vi "Initialize.vi"(8 "error in":errorcluster, 10 "parameters":variant, 11 "node in":refnum<class "BuckBoost editor node.lvclass">) -> (0 "error out":errorcluster, 2 "summary":T2[](array[typedef]), 3 "data value reference":T1)   [LabVIEW 2017, in "BuckBoost editor node.lvclass"]
doc: "Initializes the data of a node to its default state.\nThe object is not created inside of this VI, because it is created from a File depending on user selection."
uses:
  BuckBoost editor node.lvclass
  C:/Program Files (x86)/National Instruments/LabVIEW 2017/vi.lib/NI/Configuration Framework/Node/NISE_CEF_Node.lvclass
  <vilib>/NI/Configuration Framework/Node/Summary.ctl
  <vilib>/NI/Configuration Framework/Node/NodeRef.ctl
  <vilib>/NI/Configuration Framework/Node/NISE_CEF_Node.lvclass
  module/configuration/BuckBoost configuration.lvclass
  C:/Program Files (x86)/National Instruments/LabVIEW 2017/vi.lib/NI/Configuration Framework/serializable configuration/NISE_CEF_serializable configuration.lvclass
  <vilib>/NI/PowerElectronicsControl/Buck-Boost/RealTime/modulationConfig.ctl
  <vilib>/NI/PowerElectronicsControl/Buck-Boost/RealTime/TuningParameters.ctl
  <vilib>/rvi/Analysis/control/PID/Typedef/niFpgaPID_PIGains.ctl
  <vilib>/NI/PowerElectronicsControl/Buck-Boost/FPGA/contState.ctl
  module/configuration/BuckBoost configuration.lvclass/BuckBoost configuration.ctl
  module/configuration/Write numOfInterleaves.vi
  module/configuration/Write TuningParameters.vi
  module/configuration/Write modulationConfig.vi
  <vilib>/NI/DCAF/Tag Editor Core/control module/editor node/control module editor.lvclass
  <vilib>/NI/Configuration Framework/serializable configuration/NISE_CEF_serializable configuration.lvclass
  <vilib>/NI/PowerElectronicsControl/Buck-Boost/RealTime/BuckBoostInterface.lvlib
  <vilib>/NI/PowerElectronicsControl/Buck-Boost/FPGA/BuckBoost.lvlib
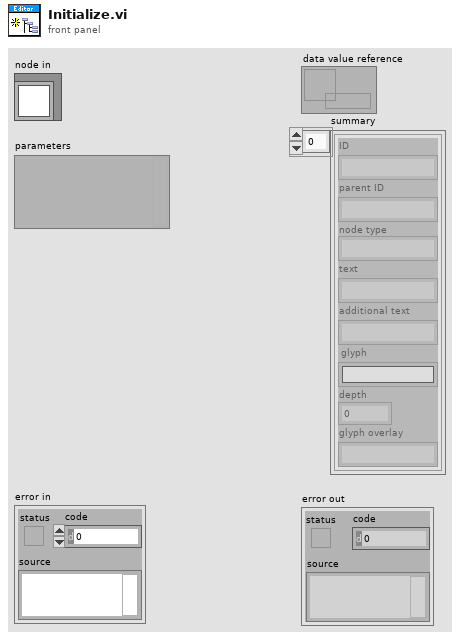
[diagram p1: front panel]
types:
  T1 = typedef "NISE_CEF_Node.lvclass/NodeRef.ctl" = refnum<data-value>
  T2 = typedef "NISE_CEF_Node.lvclass/Summary.ctl" = cluster{"ID":string, "parent ID":string, "node type":string, "text":string, "additional text":string, "glyph":string, "depth":i32, "glyph overlay":string}
  T3 = typedef "BuckBoostInterface.lvlib/TuningParameters.ctl" = cluster{"gains":T4, "manualInput":sgl, "rampRate":sgl, "pertAmp":sgl, "pertFreq":sgl, "controlFreq":sgl, "state":T5}
  T4 = typedef "niFpgaPID_PIGains.ctl" = cluster{"proportional gain":sgl, "integral gain":sgl}
  T5 = typedef "BuckBoost.lvlib/contState.ctl" = enum16{"disabled", "manual", "normal", "perturb"}
  T6 = typedef "BuckBoostInterface.lvlib/modulationConfig.ctl" = cluster{"SwitchingSpeed":dbl, "Deadband":dbl, "modulationRate":dbl}
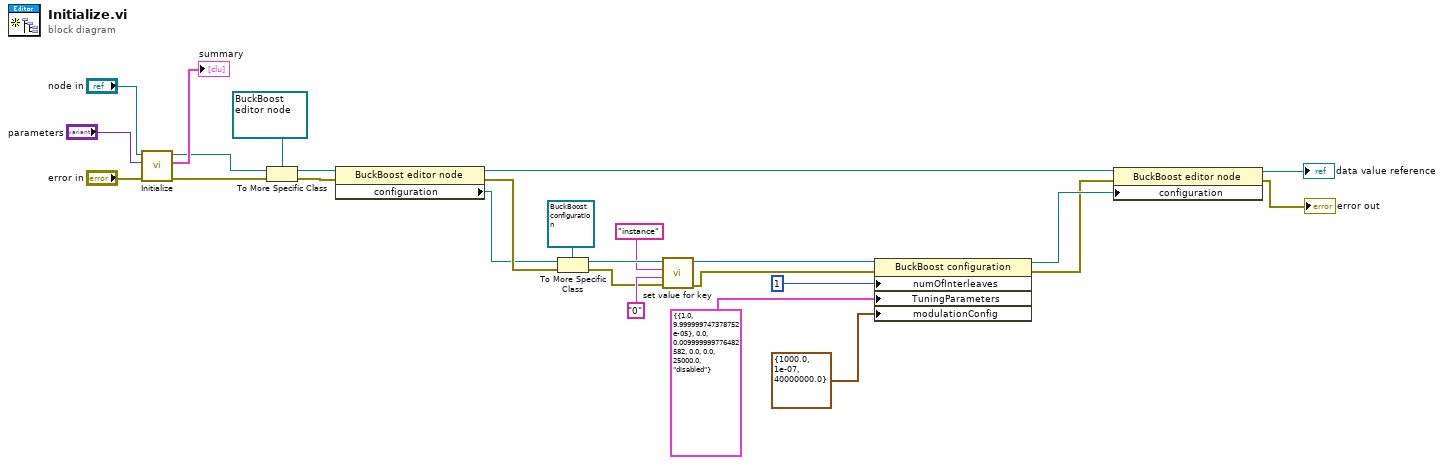
[diagram p0: block diagram]
diagram:
  n1 = call-parent "Initialize.vi"("error in"="error in", "parameters"="parameters", "node in"="node in") -> ("error out"=w22:errorcluster, "summary"=→"summary":T2[], "data value reference"=w21:T1)  [unwired: 6 in]
  n2 = To More Specific Class(target class=refnum<data-value> refnum ("data value reference"), reference=w21, error in=w22) -> (specific class reference=w19:refnum<data-value>, error out=w18:errorcluster)
  n3 = property class="BuckBoost editor node"(reference=w19, error in=w18) -> (reference out=w9:refnum<data-value>, error out=w17:errorcluster, "configuration"=w14:refnum<class "NISE_CEF_serializable configuration.lvclass">)
  n4 = To More Specific Class(target class=refnum<class "BuckBoost configuration.lvclass"> refnum ("BuckBoost configuration"), reference=w14, error in=w17) -> (specific class reference=w15:refnum<class "BuckBoost configuration.lvclass">, error out=w11:errorcluster)
  n5 = call-dynamic "set value for key.vi"("error in"=w11, "value"="0", "key"="instance", "fixed channel configuration in"=w15) -> ("error out"=w7:errorcluster, "fixed channel configuration out"=w10:refnum<class "BuckBoost configuration.lvclass">)  [unwired: 6 in]
  n6 = property class="BuckBoost configuration"(reference=w10, error in=w7, "numOfInterleaves"=u8 1, "TuningParameters"=T3 {"gains"={"proportional gain"=1.0, "integral gain"=0.0001}, "manualInput"=0.0, "rampRate"=0.01, "pertAmp"=0.0, "pertFreq"=0.0, "controlFreq"=25000.0, "state"=enum."disabled"}, "modulationConfig"=T6 {"SwitchingSpeed"=1000.0, "Deadband"=1e-07, "modulationRate"=40000000.0}) -> (reference out=w8:refnum<class "BuckBoost configuration.lvclass">, error out=w2:errorcluster)
  n7 = property class="BuckBoost editor node"(reference=w9, error in=w2, "configuration"=w8) -> (reference out=→"data value reference":refnum<data-value>, error out=→"error out":errorcluster)
